vi "SCP_Header.vi"() -> (3 "Header Output":string)   [LabVIEW 2018, in "SCP.lvlib"]
uses:
  SCP.lvlib
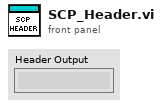
[diagram p1: front panel]
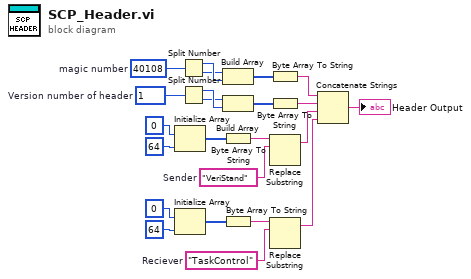
[diagram p0: block diagram]
diagram:
  w23 = "TaskControl"  # Reciever
  w18 = "VeriStand"  # Sender
  w12 = u16 1  # Version number of header
  w13 = u16 40108  # magic number
  n1 = Initialize Array(u8 0, 64 ("dimension size")) -> (w15:u8[])
  n2 = Initialize Array(u8 0, 64 ("dimension size")) -> (w21:u8[])
  n3 = Split Number(x=w13) -> (hi(x)=w6:u8, lo(x)=w5:u8)
  n4 = Split Number(x=w12) -> (hi(x)=w4:u8, lo(x)=w3:u8)
  n5 = Build Array(w5, w6) -> (w10:u8[])
  n6 = Build Array(w3, w4) -> (w11:u8[])
  n7 = Byte Array To String(unsigned byte array=w15) -> (string=w17:string)
  n8 = Byte Array To String(unsigned byte array=w21) -> (string=w19:string)
  n9 = Byte Array To String(unsigned byte array=w10) -> (string=w9:string)
  n10 = Byte Array To String(unsigned byte array=w11) -> (string=w8:string)
  n11 = Replace Substring(4:w18, 5:w17) -> (1:w2:string)  [unwired: 2 in, 1 out]
  n12 = Replace Substring(4:w23, 5:w19) -> (1:w1:string)  [unwired: 2 in, 1 out]
  n13 = Concatenate Strings(w9, w8, w2, w1) -> (→"Header Output":string)
